vi "Check Data_.vi"(11 "Mean Prefiltered Signals":dbl[](array[numeric])=[133.12, 30.72, 92.16, 450.56, 163.84, 235.52, 71.68, 112.64, 51.2, 0.0, -163.84, -102.4, -20.48, 92.16, 215.04, 184.32, 102.4, 266.24, -71.68, 10.24, -153.6, -10.24, 51.2, 266.24, -30.72, 296.96, -194.56, 163.84, -81.92, 10.24, 20.48, 102.4, -61.44, 92.16, 143.36, 92.16, 40.96, -51.2, 235.52, 153.6, 143.36, 30.72, 40.96, 235.52, -40.96, -92.16, 194.56, 184.32, -40.96, 153.6, 61.44, -71.68, -61.44, -20.48, 102.4, -133.12, 256.0, 81.92, 184.32, 215.04, 10.24, -40.96, 81.92, 266.24, -30.72, 122.88, -61.44, -30.72, 122.88, 61.44, -61.44, 102.4, -51.2, 0.0, 71.68, 225.28, 102.4, 112.64, 92.16, 225.28, 10.24, -30.72, 133.12, 81.92, 81.92, 51.2, 153.6, 20.48, 122.88, 235.52, 133.12, 225.28, 163.84, -81.92, 143.36, -20.48, -20.48, 133.12, -92.16, -51.2, 112.64, 163.84, 0.0, 317.44, 81.92, -40.96, 378.88, -10.24, 163.84, -81.92, 184.32, 51.2, 92.16, 20.48, 133.12, -10.24, 20.48, 184.32, 40.96, 163.84, -20.48, 112.64, 20.48, 20.48, 81.92, 40.96, -102.4, 102.4, 225.28, 276.48, 358.4, -20.48, 51.2, 61.44, 235.52, 286.72, -61.44, 133.12, 51.2, 30.72, 133.12, 81.92, 92.16, 163.84, 614.4, 174.08, 143.36, 71.68, 40.96, 174.08, 92.16, 143.36, 143.36, 194.56, 276.48, -51.2, 245.76, 30.72, 409.6, -225.28, 133.12, -133.12, -71.68, 194.56, -102.4, 225.28, -286.72, -81.92, -143.36, -153.6, 174.08, -71.68, -51.2, 92.16, -10.24, 102.4, 163.84, -30.72, 40.96, 20.48, 245.76, 71.68, -20.48, 204.8, -10.24, 122.88, 194.56, 102.4, 215.04, -71.68, 20.48, 92.16, 266.24, -215.04, 133.12, -10.24, 71.68, 245.76, 143.36, 0.0, 51.2, 174.08, 235.52, 235.52, 153.6, 30.72, 61.44, 235.52, -133.12, 399.36, 102.4, 40.96, 266.24, 102.4, 174.08, 92.16, 317.44, 358.4, 0.0, 20.48, 81.92, -143.36, 245.76, 10.24, -10.24, 409.6, 20.48, 51.2, -286.72, -51.2, 30.72, 30.72, -163.84, 327.68, 61.44, -194.56, 81.92, -40.96, -112.64, 174.08, 30.72, -102.4, -122.88, 184.32, 8570.88, 235.52, 4956.16, 3399.68, 4638.72, 3901.44, 4106.24, 4290.56, 3543.04, 4782.08, 419.84, 8212.48, 3768.32, 4536.32, 3860.48, 4198.4, 3962.88, 4311.04, 4771.84, 3727.36, 4444.16, 4454.4, 3880.96, 4556.8, 481.28, 8243.2, 4556.8, 3461.12, 3256.32, 4823.04, 8048.64, 348.16, 3747.84, 4177.92, 6092.8, 2017.28, 2058.24, 6502.4, 4321.28, 4188.16, 4044.8, 4157.44, 4270.08, 4270.08, 4106.24, 4372.48, 4341.76, 4024.32, 4208.64, 4198.4, 4689.92, 4259.84, 4259.84, 4116.48, 4116.48, 4229.12, 4341.76, 4167.68, 3747.84, 4372.48, 4055.04, 4014.08, 3942.4, 4065.28, 6410.24, 1935.36, 4034.56, 4167.68, 3563.52, 4638.72, 4771.84, 3164.16, 4669.44, 3911.68, 3215.36, 5160.96, 1792.0, 6420.48, 4259.84, 4300.8, 4157.44, 4003.84, 4239.36, 4024.32, 3921.92, 4618.24, 4126.72, 4177.92, 2017.28, 6666.24, 4065.28, 4259.84, 4720.64, 3645.44, 3031.04, 5130.24, 3512.32, 4751.36, 5089.28, 3215.36, 6420.48, 1884.16, 4362.24, 4300.8, 4372.48, 4126.72, 2140.16, 6799.36, 6164.48, 2170.88, 3860.48, 4188.16, 4044.8, 4034.56, 3911.68, 4014.08, 4147.2, 4106.24, 4034.56, 4362.24, 4177.92, 4157.44, 4167.68, 4085.76, 3870.72, 4464.64, 4648.96, 4085.76, 4055.04, 4126.72, 4065.28, 4198.4, 5068.8, 3051.52, 4167.68, 3819.52, 3225.6, 5652.48, 3665.92, 4362.24, 3840.0, 4106.24, 4188.16, 4055.04, 4055.04, 4208.64, 4147.2, 4044.8, 3993.6, 4126.72, 4116.48, 3799.04, 4024.32, 4085.76, 4034.56, 4352.0, 4157.44, 4259.84, 3962.88, 4177.92, 3942.4, 4014.08, 4116.48, 4218.88, 3952.64, 4208.64, 4311.04, 4096.0, 4075.52, 4106.24, 4198.4, 4198.4, 4290.56, 4188.16, 3901.44, 4423.68, 4055.04, 4188.16, 4014.08, 4280.32, 3983.36, 4321.28, 4044.8, 4075.52, 4024.32, 4136.96, 4126.72, 4096.0, 4055.04, 4382.72, 4106.24, 4249.6, 4024.32, 4198.4, 4065.28, 4055.04, 4167.68, 4096.0, 3973.12, 4096.0, 4167.68, 4126.72, 3983.36, 4341.76, 4075.52, 4311.04, 4085.76, 4096.0, 3880.96, 4177.92, 4403.2, 4055.04, 4270.08, 4085.76, 4044.8, 3829.76, 4044.8, 4280.32, 4126.72, 4024.32, 4065.28, 4055.04, 3901.44, 4321.28, 4065.28, 4331.52, 4157.44, 4188.16, 4126.72, 4423.68, 4157.44, 4218.88, 4126.72, 4249.6, 4106.24, 4044.8, 3962.88, 4249.6, 4126.72, 4270.08, 5089.28, 3215.36, 4014.08, 4208.64, 4218.88, 4116.48, 4055.04, 4362.24, 3921.92, 4331.52, 4474.88, 3993.6, 4669.44, 3491.84, 4177.92, 4147.2, 4208.64, 3932.16, 3952.64, 4474.88, 3665.92, 4823.04, 4259.84, 4096.0, 3246.08, 5232.64, 4024.32, 4321.28, 4382.72, 4157.44, 4116.48, 3993.6, 3952.64, 4096.0, 3962.88, 4423.68, 4761.6, 3778.56, 4136.96, 4034.56, 3276.8, 4751.36, 3901.44, 4280.32, 4116.48, 3901.44, 4085.76, 3942.4, 4147.2, 4280.32, 4014.08, 4106.24, 4300.8, 4065.28, 4014.08, 4075.52, 4249.6, 4157.44, 4188.16, 4270.08, 4157.44, 4290.56, 4096.0, 4392.96, 4167.68, 4259.84, 4311.04, 4106.24, 4055.04, 4249.6, 4321.28, 4188.16, 3942.4, 4188.16, 4147.2, 4280.32, 4147.2, 4136.96, 4157.44, 4352.0, 4147.2, 4331.52, 4085.76, 4362.24, 4229.12, 4085.76, 4044.8, 4096.0, 4096.0, 4352.0, 4188.16, 4188.16, 4034.56, 4321.28, 4075.52, 3983.36, 3215.36, 5304.32, 4096.0, 4147.2, 3799.04, 4208.64, 4157.44, 4198.4, 4280.32, 4229.12, 4055.04, 4352.0, 3819.52, 4782.08, 4239.36, 4382.72, 3932.16, 4546.56, 4382.72, 3901.44, 4802.56, 3747.84, 4126.72, 4280.32, 5120.0, 3450.88, 4259.84, 4239.36, 4198.4, 4024.32, 4208.64, 4485.12, 4126.72, 4126.72, 4362.24, 3809.28, 3563.52, 4741.12, 3973.12, 4648.96, 4546.56, 3655.68, 4270.08, 4014.08, 3880.96, 4311.04, 3932.16, 4423.68, 4106.24, 4239.36, 4126.72, 4126.72, 4157.44, 4116.48, 4136.96, 3901.44, 4229.12, 4413.44, 4280.32, 4321.28, 4177.92, 4116.48, 4321.28, 4167.68, 4075.52, 4239.36, 4136.96, 3932.16, 4167.68, 3962.88, 4065.28, 4218.88, 4270.08, 4239.36, 3973.12, 4014.08, 4198.4, 3891.2, 3911.68, 4270.08, 4147.2, 4372.48, 4300.8, 3942.4, 3297.28, 5222.4, 3921.92, 4454.4, 4966.4, 3266.56, 4147.2, 4044.8, 3973.12, 4075.52, 3860.48, 4198.4, 3901.44, 4208.64, 3747.84, 4352.0, 4382.72, 4300.8, 3778.56, 4485.12, 4014.08, 4167.68, 4055.04, 4423.68, 4321.28, 4177.92, 4423.68, 4065.28, 4433.92, 4044.8, 4341.76, 4362.24, 4392.96, 4259.84, 4270.08, 4106.24, 4229.12, 4270.08, 4464.64, 4648.96, 4249.6, 4259.84, 4065.28, 4014.08, 4024.32, 4270.08, 4167.68, 4034.56, 4075.52, 4157.44, 4075.52, 4218.88, 4055.04, 4106.24, 3870.72, 4136.96, 4229.12, 4331.52, 4024.32, 4198.4, 4044.8, 4085.76, 4362.24, 4259.84, 4300.8, 4055.04, 4055.04, 4433.92, 4167.68, 4536.32, 4055.04, 4136.96, 4085.76, 4065.28, 4413.44, 4055.04, 4044.8, 4341.76, 4034.56, 4362.24, 3829.76, 4362.24, 4065.28, 4085.76, 4157.44, 4157.44, 4403.2, 4167.68, 4208.64, 4423.68, 4270.08, 4495.36, 4218.88, 4177.92, 4218.88, 4454.4, 4218.88, 4034.56, 4136.96, 4392.96, 4720.64, 3665.92, 4198.4, 4321.28, 4218.88, 3840.0, 3952.64, 4444.16, 3706.88, 4567.04, 4075.52, 4147.2, 4024.32, 4444.16, 4485.12, 4106.24, 3911.68, 4096.0, 4270.08, 4270.08, 4229.12, 4167.68, 4003.84, 4352.0, 4167.68, 4055.04, 4218.88, 4423.68, 4126.72, 4311.04, 4208.64, 4126.72, 3901.44, 4280.32, 4167.68, 4239.36, 4218.88, 4136.96, 4003.84, 4096.0, 4147.2, 4096.0, 4096.0, 3921.92, 4126.72, 4157.44, 4085.76, 4259.84, 4218.88, 4198.4, 3829.76, 3983.36, 4218.88, 4311.04, 4065.28, 4024.32, 3932.16, 4157.44, 4014.08, 4055.04, 4106.24, 4270.08, 4136.96, 4382.72, 4208.64, 4249.6, 4403.2, 4136.96, 3993.6, 4229.12, 4331.52, 4280.32, 4075.52, 4188.16, 4096.0, 4126.72, 4065.28, 4198.4, 4085.76, 4167.68, 4403.2, 3962.88, 4116.48, 4259.84, 4198.4, 4280.32, 4085.76, 4188.16, 4249.6, 4085.76, 4157.44, 4372.48, 4229.12, 4403.2, 3952.64, 4208.64, 3973.12, 4075.52, 4229.12, 4147.2, 4116.48, 4311.04, 4249.6, 4454.4, 4188.16, 4239.36, 4126.72, 4372.48, 4157.44, 4290.56, 4188.16, 4300.8, 4075.52, 4382.72, 4147.2, 4136.96, 4177.92, 4188.16, 4177.92, 4403.2, 4208.64, 4157.44, 4218.88, 4188.16, 4014.08, 4065.28, 4239.36, 4280.32, 4198.4, 4444.16, 4106.24, 4136.96, 3921.92, 4116.48, 4300.8, 4198.4, 3921.92, 4167.68, 4157.44, 4290.56, 3993.6, 4218.88, 4198.4, 4413.44, 4024.32, 4311.04, 4116.48, 4341.76, 4126.72, 4392.96, 4147.2, 4055.04, 4300.8, 3952.64, 4392.96, 4331.52, 4126.72, 4270.08, 4034.56, 4362.24, 4014.08, 4362.24, 3973.12, 4413.44, 4167.68, 4331.52, 4096.0, 4198.4, 4249.6, 4259.84, 4229.12, 4177.92, 4116.48, 4208.64, 4055.04, 4290.56, 4300.8, 4280.32, 4116.48, 4034.56, 4372.48, 4208.64, 3942.4, 4382.72, 4055.04, 4372.48, 4311.04, 4259.84, 3962.88, 4280.32, 4044.8, 4249.6, 4096.0, 4014.08, 4003.84, 4044.8, 4208.64, 4167.68, 4372.48, 4444.16, 4270.08, 4300.8, 3942.4, 4433.92, 4147.2, 4382.72, 4003.84, 4362.24, 4321.28, 4126.72, 4147.2, 4259.84, 4075.52, 4044.8, 3932.16, 4362.24, 4085.76, 4444.16, 4126.72, 4249.6, 4085.76, 3973.12, 4218.88, 4208.64, 4034.56, 4239.36, 4177.92, 4208.64, 4362.24, 4147.2, 4106.24, 4218.88, 4188.16, 4188.16, 4024.32, 4526.08, 3973.12, 4208.64, 4055.04, 4495.36, 4249.6, 4136.96, 3952.64, 4218.88, 3676.16, 4239.36, 4167.68, 4300.8, 3993.6, 4249.6, 4157.44, 3911.68, 4096.0, 4116.48, 4085.76, 4157.44, 4096.0, 4044.8, 4096.0, 4259.84, 4198.4, 4577.28, 4259.84, 4270.08, 4270.08, 4239.36, 4003.84, 4362.24, 3952.64, 4577.28, 4024.32, 4321.28, 4208.64, 4188.16, 4311.04, 4352.0, 4403.2, 4096.0, 3962.88, 4229.12, 4167.68, 4188.16, 4096.0, 4075.52, 4280.32, 4229.12, 4065.28, 4188.16, 4454.4, 4352.0, 4198.4, 4075.52, 4290.56, 4229.12, 4392.96, 4116.48, 4014.08, 3655.68, 4259.84, 4505.6, 4014.08, 4352.0, 4239.36, 4454.4, 4044.8, 4034.56, 4188.16, 4249.6, 4587.52, 4321.28, 4311.04, 4280.32, 3727.36, 4536.32, 4106.24, 4085.76, 4341.76, 4464.64, 3788.8, 4229.12, 4311.04, 4116.48, 3993.6, 4321.28, 4147.2, 4065.28, 4136.96, 4218.88, 4270.08, 4331.52, 4218.88, 4280.32, 4167.68, 4003.84, 4208.64, 4413.44, 4218.88, 4024.32, 3983.36, 4331.52, 4239.36, 4229.12, 4239.36, 4136.96, 4249.6, 4198.4, 4126.72, 4136.96, 4198.4, 4147.2, 4106.24, 4290.56, 4167.68, 4372.48, 3962.88, 4218.88, 4014.08, 4096.0, 4270.08, 4106.24, 4106.24, 4229.12, 4136.96, 4423.68, 3891.2, 4014.08, 4270.08, 4034.56, 4413.44, 4413.44, 4198.4, 4474.88, 4239.36, 4177.92, 4239.36, 4147.2, 4055.04, 4218.88, 4270.08, 4249.6, 4044.8, 4280.32, 4188.16, 4372.48, 4075.52, 4096.0, 4362.24, 4188.16, 4167.68, 4311.04, 4177.92, 4372.48, 4239.36, 4259.84, 3983.36, 4280.32, 4147.2, 4321.28, 4188.16, 4126.72, 4331.52, 4249.6, 4229.12, 4270.08, 4024.32, 4341.76, 4218.88, 3993.6, 4771.84, 3706.88, 4024.32, 4587.52, 4188.16, 4034.56, 4167.68, 4659.2, 4157.44, 4218.88, 4147.2, 4331.52, 4003.84, 4065.28, 4126.72, 4331.52, 3952.64, 4444.16, 4136.96, 4341.76, 4229.12, 4044.8, 4147.2, 4403.2, 4331.52, 4177.92, 4218.88, 4055.04, 4311.04, 4270.08, 4055.04, 4444.16, 4392.96, 4382.72, 4024.32, 4239.36, 4147.2, 4495.36, 4147.2, 4218.88, 3850.24, 4382.72, 4362.24, 4157.44, 4126.72, 4444.16, 4116.48, 4474.88, 3819.52, 4689.92, 4259.84, 4505.6, 3983.36, 4096.0, 4106.24, 4188.16, 4239.36, 4362.24, 4003.84, 4300.8, 3973.12, 4546.56, 4485.12, 4280.32, 4198.4, 4311.04, 4249.6, 4362.24, 4147.2, 4147.2, 4300.8, 4198.4, 4188.16, 4147.2, 3962.88, 4126.72, 4249.6, 4331.52, 3860.48, 4311.04, 4106.24, 4270.08, 4208.64, 4126.72, 4290.56, 4372.48, 4259.84, 4034.56, 4116.48, 4300.8, 4147.2, 4372.48, 4065.28, 4229.12, 3983.36, 4167.68, -40.96, 40.96, 20.48, 30.72, 256.0, 61.44, 163.84, 122.88, -102.4, -30.72, 276.48, 215.04, 225.28, 225.28, 40.96, 276.48, 30.72, -122.88, -81.92, 112.64, 61.44, 174.08, -30.72, 40.96, 143.36, 112.64, 174.08, 71.68, 10.24, 204.8, 81.92, 112.64, 0.0, -71.68, 184.32, 102.4, 245.76, 143.36, 184.32, 153.6, -102.4, 122.88, 122.88, -61.44, 235.52, 122.88, -61.44, -92.16, 81.92, 40.96, 40.96, -143.36, -10.24, 122.88, -235.52, 20.48, 215.04, 225.28, 20.48, -92.16, 112.64, 327.68, 235.52]) -> (3 "similar":bool)   [LabVIEW 2020]
uses:
  <vilib>/Analysis/NI_AALBase.lvlib
panel:
  out "Prefiltered Signals":dbl[](graph)
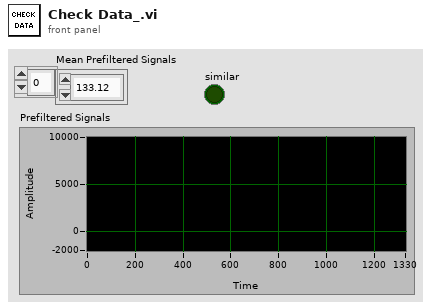
[diagram p1: front panel]
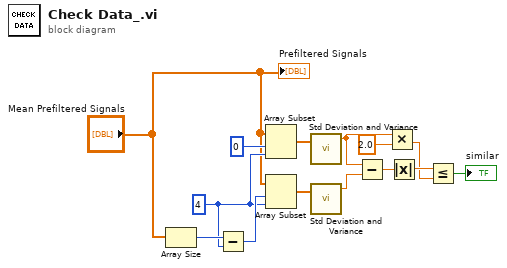
[diagram p0: block diagram]
diagram:
  w12 = 4
  n1 = Array Size(array="Mean Prefiltered Signals") -> (size(s)=w14:i32)
  n2 = Subtract(x=w14, y=w12) -> (x-y=w13:i32)
  n3 = Array Subset(array="Mean Prefiltered Signals", index=0, length=w12) -> (w10:dbl[])
  n4 = Array Subset(array="Mean Prefiltered Signals", index=w13, length=w12) -> (w9:dbl[])
  n5 = call <vilib>:"Std Deviation and Variance.vi"("X"=w10) -> ("mean"=w5:dbl)  [unwired: 1 in, 2 out]
  n6 = call <vilib>:"Std Deviation and Variance.vi"("X"=w9) -> ("mean"=w6:dbl)  [unwired: 1 in, 2 out]
  n7 = Subtract(x=w5, y=w6) -> (x-y=w8:dbl)
  n8 = Multiply(x=w5, y=2.0) -> (x*y=w2:dbl)
  n9 = Absolute Value(x=w8) -> (abs(x)=w7:dbl)
  n10 = Less Or Equal?(x=w7, y=w2) -> (x <= y?=→"similar":bool)
  "Prefiltered Signals" <- "Mean Prefiltered Signals"
